vi "Add Parameter (Double).vi"(7 "Evaluation Method (ByReference)":i32(ring)=1 items=["ByValue", "ByReference"], 8 "error in (no error)":errorcluster, 9 "Value":dbl, 10 "Identifier":string, 11 "Sequence Ref in":refnum<k24>) -> (0 "error out":errorcluster, 3 "Sequence Ref out":refnum<k24>)   [LabVIEW 2013, in "Simple Sequence Tools - Editor.lvlib"]
uses:
  Simple Sequence Tools - Editor.lvlib
  NationalInstruments.VeriStand.RealTimeSequenceDefinitionApi
  NationalInstruments.VeriStand.DataTypes
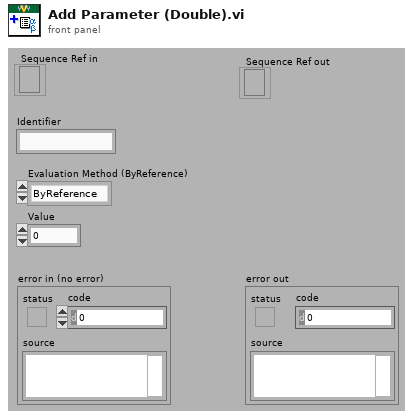
[diagram p1: front panel]
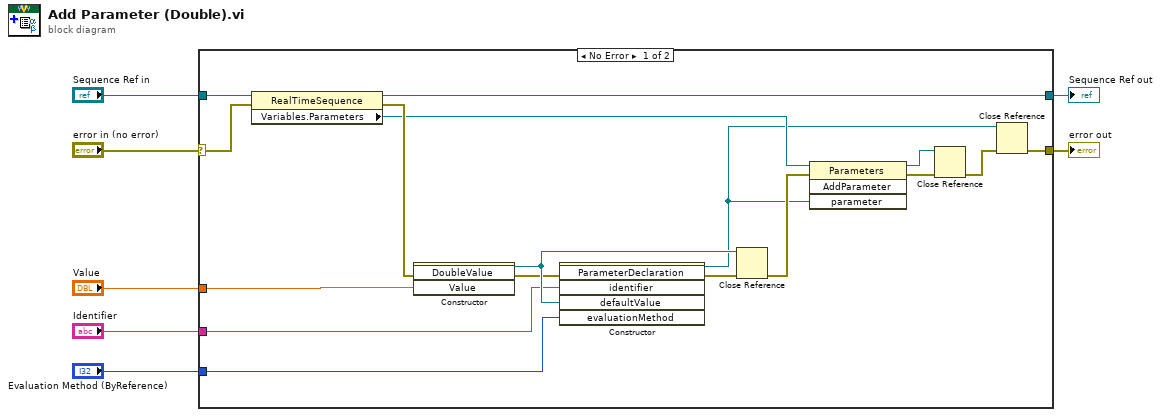
[diagram p0: block diagram]
diagram:
  n1 = case shown="No Error" "error in (no error)" {
    selector: "error in (no error)" -> [w8 w25]
    tunnel: "Value" -> [w21 _]
    tunnel: "Identifier" -> [w18 _]
    tunnel: "Evaluation Method (ByReference)" -> [w17 _]
    tunnel: "Sequence Ref in" -> [w16 w26]
    tunnel: [w15 w26] -> w3
    tunnel: [w11 w25] -> w2
    frame No Error {
      n2 = property class="RealTimeSequence"(reference=w16, error in=w8) -> (reference out=w15:refnum<k24>, error out=w20:errorcluster, "Variables.Parameters"=w19:refnum<k24>)
      n3 = constructor class="DoubleValue"(error in=w20, "Value"=w21) -> (reference out=w23:refnum<k24>, error out=w22:errorcluster)  [unwired: 2 in, 2 out]
      n4 = constructor class="ParameterDeclaration"(error in=w22, "identifier"=w18, "defaultValue"=w23, "evaluationMethod"=w17) -> (reference out=w9:refnum<k24>, error out=w14:errorcluster)  [unwired: 2 in, 4 out]
      n5 = Close Reference(reference=w23, error in (no error)=w14) -> (error out=w24:errorcluster)
      n6 = invoke class="Parameters" method="AddParameter"(reference=w19, error in=w24, "parameter"=w9) -> (reference out=w10:refnum<k24>, error out=w13:errorcluster)  [unwired: 1 in, 2 out]
      n7 = Close Reference(reference=w10, error in (no error)=w13) -> (error out=w12:errorcluster)
      n8 = Close Reference(reference=w9, error in (no error)=w12) -> (error out=w11:errorcluster)
    }
    frame Error {
    }
  }
  "Sequence Ref out" <- w3
  "error out" <- w2
